vi "Display_Temp.vi"() -> ()   [LabVIEW 2024]
uses:
  <vilib>/Utility/file.llb/Write Delimited Spreadsheet (DBL).vi
panel:
  in  "file path (dialog if empty)":path
  in  "STOP":bool
  out "Gradi Centrigradi OUT":dbl
  out "Waveform Chart":dbl(graph)
  out "Temp (F)":dbl(slide) scale=0.0..110.0
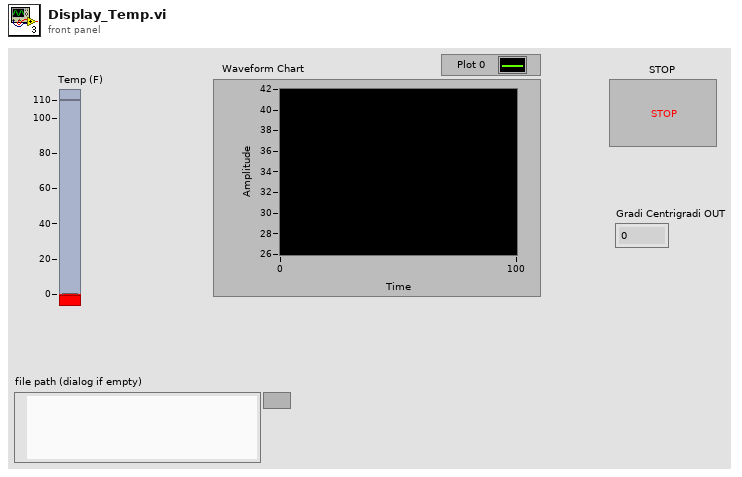
[diagram p1: front panel]
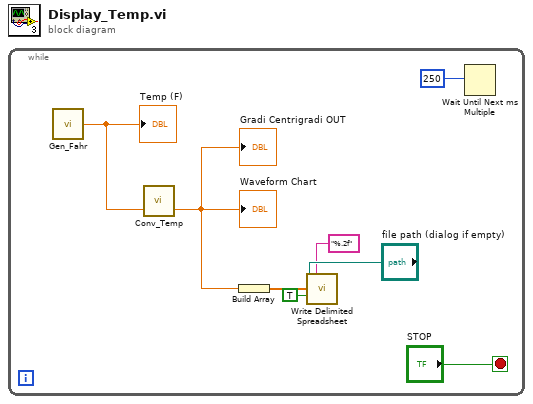
[diagram p0: block diagram]
diagram:
  n1 = while {
    stop <- "STOP" stop-if-true
    n2 = call "Gen_Fahr.vi"() -> ("Temp (F)"=w8:dbl)  [unwired: 1 in]
    "Temp (F)" <- w8
    n3 = call "Conv_Temp.vi"("Gradi Fahrenheit IN"=w8) -> ("Gradi Centrigradi OUT"=w5:dbl)  [unwired: 1 in, 1 out]
    "Waveform Chart" <- w5
    "Gradi Centrigradi OUT" <- w5
    n4 = Build Array(w5) -> (w4:dbl[])
    n5 = call-poly <vilib>:"Write Delimited Spreadsheet.vi"("file path (dialog if empty)"="file path (dialog if empty)", "format (%.3f)"="%.2f", "1D data"=w4, "append to file? (new file:F)"=TRUE) -> ()  [unwired: 10 in, 2 out]
    n6 = Wait Until Next ms Multiple(millisecond multiple=250) -> ()  [unwired: 1 out]
  }
